vi "Q4.vi"() -> ()   [LabVIEW 2020]
uses:
  <vilib>/Utility/file.llb/Read Delimited Spreadsheet (DBL).vi
panel:
  out "Average Photon Energy Ev":dbl
  in  "file path (dialog if empty)":path
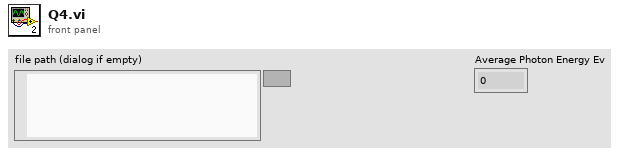
[diagram p1: front panel]
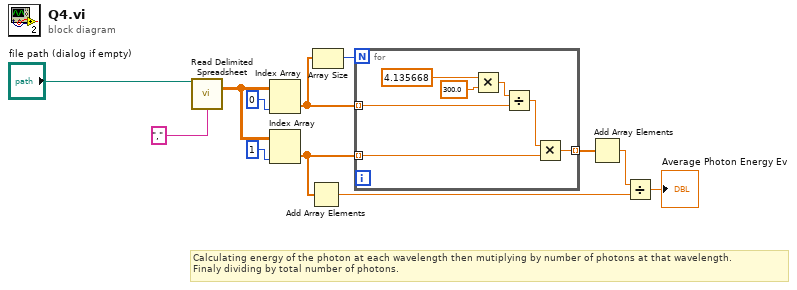
[diagram p0: block diagram]
diagram:
  # "Calculating energy of the photon at each wavelength then mutiplying by number of photons at that wavelength.\nFinaly dividing by total number of photons."
  n1 = call-poly <vilib>:"Read Delimited Spreadsheet.vi"("file path (dialog if empty)"="file path (dialog if empty)", "delimiter (\\t)"="," ("delimiter (\\t)")) -> ("all rows"=w8:dbl[][])  [unwired: 8 in, 5 out]
  n2 = Index Array(array=w8, index (col)=0 ("disabled index (col)")) -> (element=w6:dbl[])  [unwired: 1 in]
  n3 = Index Array(array=w8, index (col)=1 ("disabled index (col)")) -> (element=w5:dbl[])  [unwired: 1 in]
  n4 = Add Array Elements(numeric array=w5) -> (sum=w2:dbl)
  n5 = Array Size(array=w6) -> (size(s)=w9:i32)
  n6 = for {
    N: w9 -> [_]
    tunnel: w5 -> [w14] mode=indexing
    tunnel: w6 -> [w17] mode=indexing
    tunnel: [w13] -> w4 mode=indexing
    n7 = Multiply(x=4.135668, y=300.0) -> (x*y=w18:dbl)
    n8 = Divide(x=w18, y=w17) -> (x/y=w15:dbl)
    n9 = Multiply(x=w15, y=w14) -> (x*y=w13:dbl)
  }
  n10 = Add Array Elements(numeric array=w4) -> (sum=w3:dbl)
  n11 = Divide(x=w3, y=w2) -> (x/y=→"Average Photon Energy Ev":dbl)
